vi "Fetch Multiple Record Multiple Channel (DBL).vi"(5 "FIFO Type":T1=enum."Fast FIFO", 7 "Timeout (s)":i32=5, 8 "error in":errorcluster, 10 "Records to Fetch":i32, 11 "FPGA VI Reference In":refnum<k20>) -> (0 "error out":errorcluster, 2 "Acquired Data":dbl[][](array[numeric]) format="%.2f", 3 "FPGA VI Reference Out":refnum<k20>, 4 "Elements Remaining":u32)   [LabVIEW 2012]
uses:
  <userlib>/FlexRIO Host Library/FlexRIO Host API/Acquire/FIFO Type.ctl
  <userlib>/FlexRIO Host Library/FlexRIO Host API/Acquire/Fetch/Fetch Acquired Data (I16).vi
  <vilib>/Utility/error.llb/Error Cluster From Error Code.vi
  <vilib>/rvi/errors/niLvFpgaAdjustHostInterfaceError.vi
  <vilib>/rvi/interface/nirviReadWriteControl/nirviReadWriteControl.xnode
  NiFpgaLv.dll
  <vilib>/rvi/interface/Simulation/niFpgaSimulationCallBeginRW.vi
  <userlib>/FlexRIO Host Library/FlexRIO Host Library (User).lvlib
panel:
  out "Samples Requested":i32
  in  "Packed Samples per Cycle":i32=2
  in  "Number of Channels":i32=2
  out "Data Acquired":i16[](array[numeric])
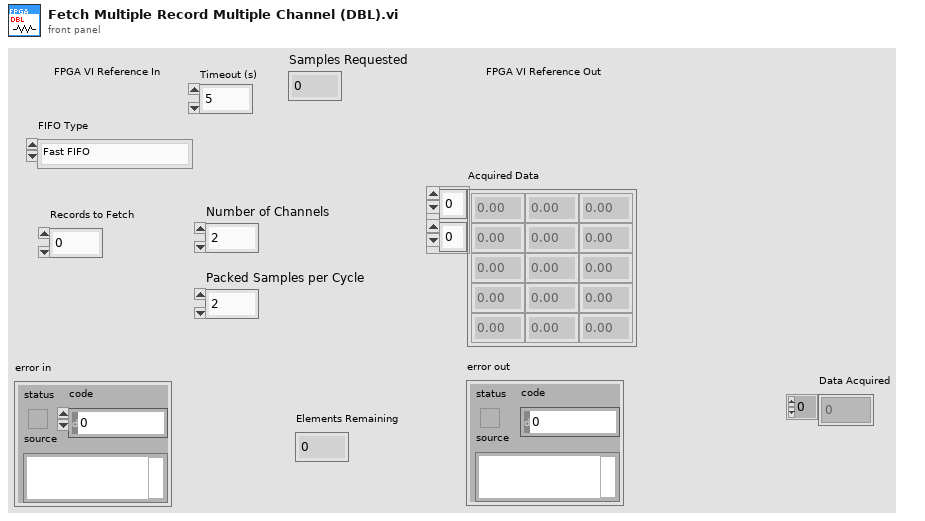
[diagram p1: front panel]
types:
  T1 = typedef "FIFO Type.ctl" = enum16{"FPGA to Host FIFO (U64)", "Generic", "FPGA to Host FIFO (U32)", "Fast FIFO"}
  T2 = cluster{"Load Record Parameters?":bool, "Pre Trigger Samples":u16, "Samples per Record":u16, "Trigger Hold Off":u16, "Record Count":u16}
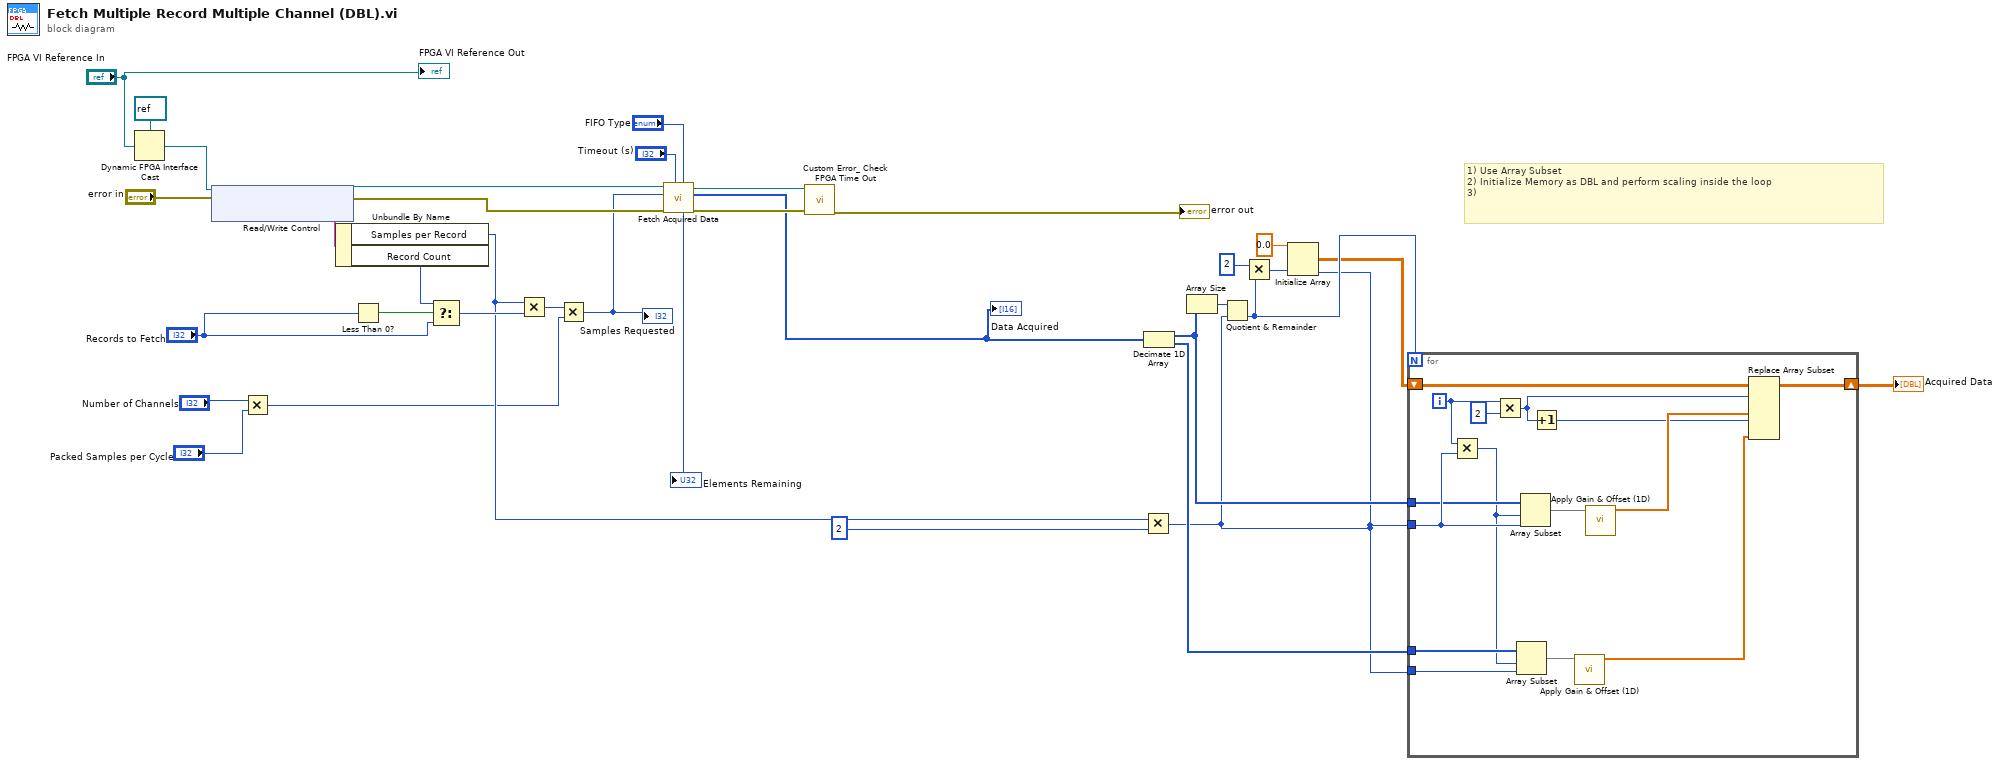
[diagram p0: block diagram]
diagram:
  # "1) Use Array Subset\n2) Initialize Memory as DBL and perform scaling inside the loop\n3)"
  n1 = Dynamic FPGA Interface Cast(Session In=refnum<k20> refnum ("Type"), Type="FPGA VI Reference In") -> (Session Out=w32:refnum<k20>)
  n2 = xnode "Read/Write Control"("FPGA VI Reference In"=w32, "error in"="error in") -> ("FPGA VI Reference Out"=w27:refnum<k20>, "error out"=w26:errorcluster, "Record Parameters"=w31:T2)
  n3 = Multiply(x="Number of Channels", y="Packed Samples per Cycle") -> (x*y=w2:i32)
  n4 = Unbundle By Name(w31) -> ("Samples per Record"=w22:u16, "Record Count"=w29:u16)
  n5 = Less Than 0?(x="Records to Fetch") -> (x < 0?=w30:bool)
  n6 = Select(t=w29, s=w30, f="Records to Fetch") -> (s? t:f=w23:i32)
  n7 = Multiply(x=w22, y=w23) -> (x*y=w3:i32)
  n8 = Multiply(x=w3, y=w2) -> (x*y=w1:i32)
  "Samples Requested" <- w1
  n9 = call-poly <userlib>:"Fetch Acquired Data.vi"("FIFO Type"="FIFO Type", "Timeout (s)"="Timeout (s)", "error out"=w26, "Samples"=w1, "FPGA Reference In"=w27) -> ("error out"=w17:errorcluster, "Data"=w7:i16[], "FPGA Reference Out"=w18:refnum<k20>, "Elements Remaining"=→"Elements Remaining":u32)  [unwired: 3 in]
  "Data Acquired" <- w7
  n10 = call <userlib>:"Custom Error_ Check FPGA Time Out.vi"("error in"=w17, "FPGA VI Reference In"=w18) -> ("error out"=→"error out":errorcluster)  [unwired: 8 in, 1 out]
  n11 = Multiply(x=w22, y=u16 2) -> (x*y=w10:u16)
  n12 = Decimate 1D Array(w7) -> (w20:i16[], w11:i16[])
  n13 = Array Size(array=w20) -> (size(s)=w19:i32)
  n14 = Quotient & Remainder(x=w19, y=w10) -> (floor(x/y)=w14:i32)  [unwired: 1 out]
  n15 = Multiply(x=2, y=w14) -> (x*y=w15:i32)
  n16 = Initialize Array(0.0 ("element"), w15, w10) -> (w12:dbl[][])
  n17 = for {
    N: w14 -> [_]
    tunnel: w20 -> [w49]
    tunnel: w10 -> [w50]
    tunnel: w11 -> [w48]
    tunnel: w10 -> [w46]
    shift-right: [w44] -> w9
    shift-left: w12 -> [w45]
    i -> [w41]
    n18 = Multiply(x=w41, y=w50) -> (x*y=w47:i32)
    n19 = Multiply(x=w41, y=2) -> (x*y=w39:i32)
    n20 = Array Subset(array=w48, index=w47, length=w46) -> (w42:i16[])
    n21 = Array Subset(array=w49, index=w47, length=w50) -> (w43:i16[])
    n22 = Increment(x=w39) -> (x+1=w37:i32)
    n23 = call <userlib>:"Apply Gain & Offset (1D).vi"("Raw Data"=w42) -> ("Scaled Data"=w36:dbl[])  [unwired: 10 in]
    n24 = call <userlib>:"Apply Gain & Offset (1D).vi"("Raw Data"=w43) -> ("Scaled Data"=w38:dbl[])  [unwired: 10 in]
    n25 = Replace Array Subset(array=w45, new element #1=w38, index (row) #1=w39, new element #2=w36, index (row) #2=w37) -> (w44:dbl[][])  [unwired: 2 in]
  }
  "Acquired Data" <- w9
  "FPGA VI Reference Out" <- "FPGA VI Reference In"
